vi "Make circle bounding rectangle.vi"(1 "circle radius":i32, 2 "Coordinates":cluster{i32, i32}) -> (0 "Bounding Rectangle":T1)   [LabVIEW 2016]
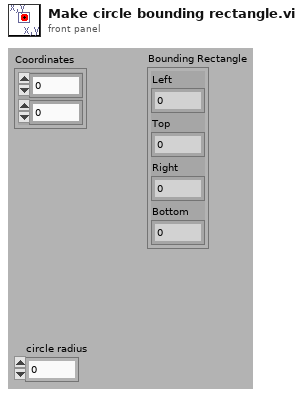
[diagram p1: front panel]
types:
  T1 = cluster{"Left":i32, "Top":i32, "Right":i32, "Bottom":i32}
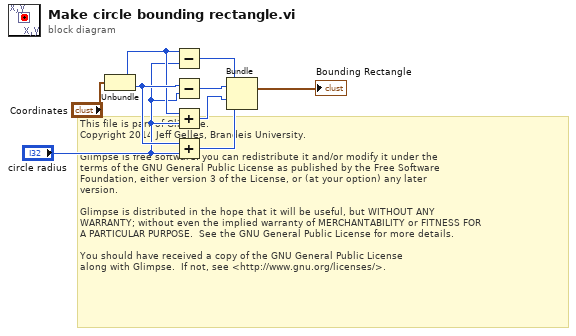
[diagram p0: block diagram]
diagram:
  # "This file is part of Glimpse. \nCopyright 2014 Jeff Gelles, Brandeis University.    \n\nGlimpse is free software: you can redistribute it and/or modify it under the \nterms of the GNU General Public License as published by the Free Software \nFoundation, either version 3 of the License, or (at your option) any later \nversion.\n\nGlimpse is distributed in the hope that it will be useful, but WITHOUT ANY \nWARRANTY; without even the implied warranty of MERCHANTABILITY or FITNESS FOR \nA PARTICULAR PURPOSE.  See the GNU General Public License for more details.\n\nYou should have received a copy of the GNU General Public License\nalong with Glimpse.  If not, see <http://www.gnu.org/licenses/>."
  n1 = Unbundle("Coordinates") -> (w7:i32, w8:i32)
  n2 = Subtract(x=w7, y="circle radius") -> (x-y=w3:i32)
  n3 = Subtract(x=w8, y="circle radius") -> (x-y=w4:i32)
  n4 = Add(x=w7, y="circle radius") -> (x+y=w5:i32)
  n5 = Add(x=w8, y="circle radius") -> (x+y=w2:i32)
  n6 = Bundle(w3, w4, w5, w2) -> (→"Bounding Rectangle":cluster{i32, i32, i32, i32})  [unwired: 1 out]
